vi "hse-application_DetermineProgramPaths.vi"(8 "error in":errorcluster, 11 "Application in":refnum<class "hse-application.lvclass">) -> (0 "error out":errorcluster, 3 "Application out":refnum<class "hse-application.lvclass">)   [LabVIEW 2020, in "hse-application.lvclass"]
doc: "Determines the Application Base, Configuration and Data paths.\n____\nHAMPEL SOFTWARE ENGINEERING v3.8.0 (2023-12-18 14:41)"
uses:
  hse-application.lvclass
  hse-application.lvclass/hse-application.ctl
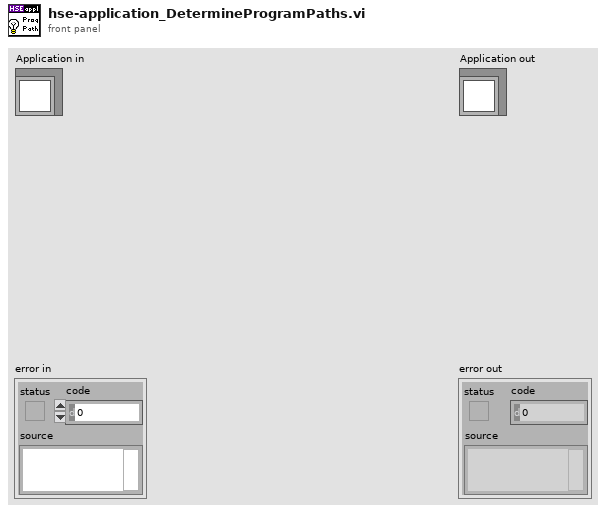
[diagram p1: front panel]
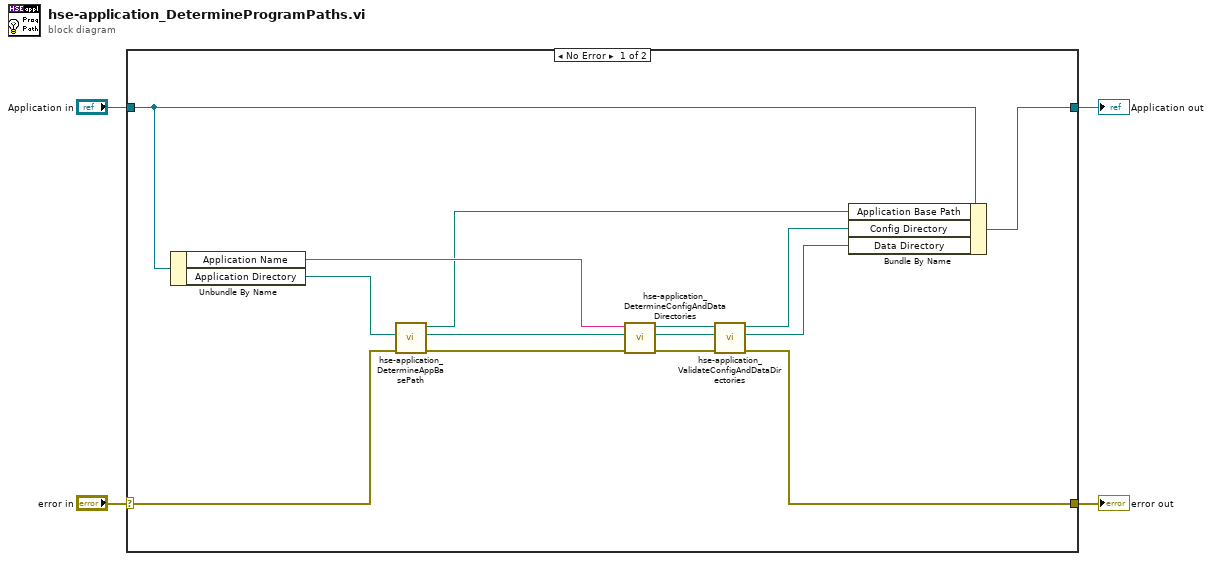
[diagram p0: block diagram]
diagram:
  n1 = case shown="No Error" "error in" {
    selector: "error in" -> [w10 w19]
    tunnel: [w14 w19] -> w3
    tunnel: [w16 w20] -> w1
    tunnel: "Application in" -> [w18 w20]
    frame No Error {
      n2 = Unbundle By Name(w18) -> ("Application Name"=w6:string, "Application Directory"=w8:path)
      n3 = call "hse-application_DetermineAppBasePath.vi"("error in"=w10, "Application Directory"=w8) -> ("error out"=w9:errorcluster, "Application Directory DUP"=w7:path, "App Base Path"=w5:path)  [unwired: 7 in]
      n4 = call "hse-application_DetermineConfigAndDataDirectories.vi"("error in"=w9, "Application Directory"=w7, "Application Name"=w6) -> ("error out"=w11:errorcluster, "Data Directory"=w12:path, "Config Directory"=w13:path)  [unwired: 6 in]
      n5 = call "hse-application_ValidateConfigAndDataDirectories.vi"("error in (no error)"=w11, "Data Directory"=w12, "Config Directory"=w13) -> ("error out"=w14:errorcluster, "Data Directory DUP"=w15:path, "Config Directory DUP"=w17:path)  [unwired: 6 in]
      n6 = Bundle By Name(cluster=w18, "Application Base Path"=w5, "Config Directory"=w17, "Data Directory"=w15) -> (w16:refnum<class "hse-application.lvclass">)
    }
    frame Error {
    }
  }
  "error out" <- w3
  "Application out" <- w1
